vi "Flow Sensors Control.vi"(5 "Initialized Array Cluster":T3, 7 "Initialized Index":i32, 9 "Apply Savitsky-Golay?":bool, 11 "Slave Data Cluster":T1={"Current DoE"=[], "SSI 1 Flow Rate"=0.0, "SSI 2 Flow Rate"=0.0, "FLOM 1 Flow Rate"=0.0, "FLOM 2 Flow Rate"=0.0, "Pumps Running?"=FALSE, "Boolean 2"=FALSE, "Boolean 3"=FALSE, "Boolean 4"=FALSE, "At Equilibrium?"=FALSE, "Script Running?"=FALSE, "Current Script Iteration"=0.0, "Total Script Iterations"=0.0, "FLOM Pumps VISA"="COM2", "SSI 1 Pump VISA"="COM76", "SSI 2 Pump VISA"="COM74", "Huber Unistat VISA"="COM1", "SSI 3 Pump VISA"="COM76", "SSI 4 Pump VISA"="COM76", "SSI 4 Flow Rate"=0.0, "SSI 3 Flow Rate"=0.0, "Flow Meter 1 Rate "=0.0, "Flow Meter 2 Rate"=0.0, "Flow Meter 3 Rate"=0.0, "Flow Meter 4 Rate"=0.0, "SSI 1 Flow Setpoint"=0.0, "SSI 2 Flow Setpoint"=0.0, "SSI 3 Flow Setpoint"=0.0, "SSI 4 Flow Setpoint"=0.0, "Temperature Setpoint"=0.0, "Flow meter 3 COM"=17, "Flow meter 5 COM"=18, "Flow meter 4 COM"=19, "Flow meter 2 COM"=16, "Flow meter 1 COM"=15, "Unit"=enum."PSI", "Pressure COM"="COM6", "Julabo Setpoint"=0.0, "Julabo Control"=enum."Internal", "Overtemp"=50.0, "Subtemp"=-20.0, "HeatMax"=50, "CoolMax"=-100, "InternMax"=50.0, "InternMin"=0.0, "Upper Bandlimit"=100.0, "Lower Bandlimit"=0.0, "Julabo CF41 VISA"="COM3", "Xp (0.6K) Int"=0.6, "Tn (3s) Int"=3, "Tv (0s) Int"=0, "Dynamic (0: aperiodic) Int"=enum."aperiodic", "Xp (0.6K) Ext"=0.6, "Tn (3s) Ext"=3, "Tv (0s) Ext"=0, "XpU (0.6K) Ext"=0.6, "Julabo Serial Configuration"={"Baud Rate"=4800, "Parity"=2, "Data Bits"=7, "Stop Bits"=10, "Flow Control"=2}} {"Julabo Serial Configuration"."Flow Control" items=["None", "XON/XOFF", "RTS/CTS", "XON/XOFF & RTS/CTS", "DTR/DSR", "XON/XOFF & DTR/DSR"]; "Julabo Serial Configuration"."Stop Bits" items=["1.0"=10, "1.5"=15, "2.0"=20]; "Julabo Serial Configuration"."Data Bits" items=["7"=7, "8"=8]; "Julabo Serial Configuration"."Parity" items=["None", "Odd", "Even", "Mark", "Space"]; "Julabo Serial Configuration"."Baud Rate" items=["300"=300, "600"=600, "1200"=1200, "2400"=2400, "4800"=4800, "9600"=9600, "19200"=19200]; "XpU (0.6K) Ext" min=0.1 max=99.9; "Tv (0s) Ext" max=999; "Tn (3s) Ext" min=3 max=9999; "Xp (0.6K) Ext" min=0.1 max=99.9; "Tv (0s) Int" max=999; "Tn (3s) Int" min=3 max=9999; "Xp (0.6K) Int" min=0.1 max=99.9; "Lower Bandlimit" min=0.0 max=200.0; "Upper Bandlimit" min=0.0 max=200.0; "InternMin" format="%.2f"; "InternMax" format="%.2f"; "CoolMax" min=-100 max=0; "HeatMax" max=100; "Subtemp" format="%.2f"; "Overtemp" format="%.2f"; "Julabo Setpoint" format="%.2f"; "Current DoE" format="%0.3f"}) -> (1 "Flow Rate Data Out":cluster{dbl, dbl, dbl, dbl, dbl}, 2 "Numeric out":i32, 3 "Flow Rate Data Array Cluster Out":T3)   [LabVIEW 2015]
uses:
  --Controls and TypeDefs--/DoE_Control_Cluster.ctl
  <instrlib>/JULABO DeviceDriver/Examples/Julabo Serial Control.ctl
  <vilib>/ptbypt/NI_PtbyPt.lvlib
panel:
  # "Julabo"
  # "Limits"
  # "PID Control Parameters"
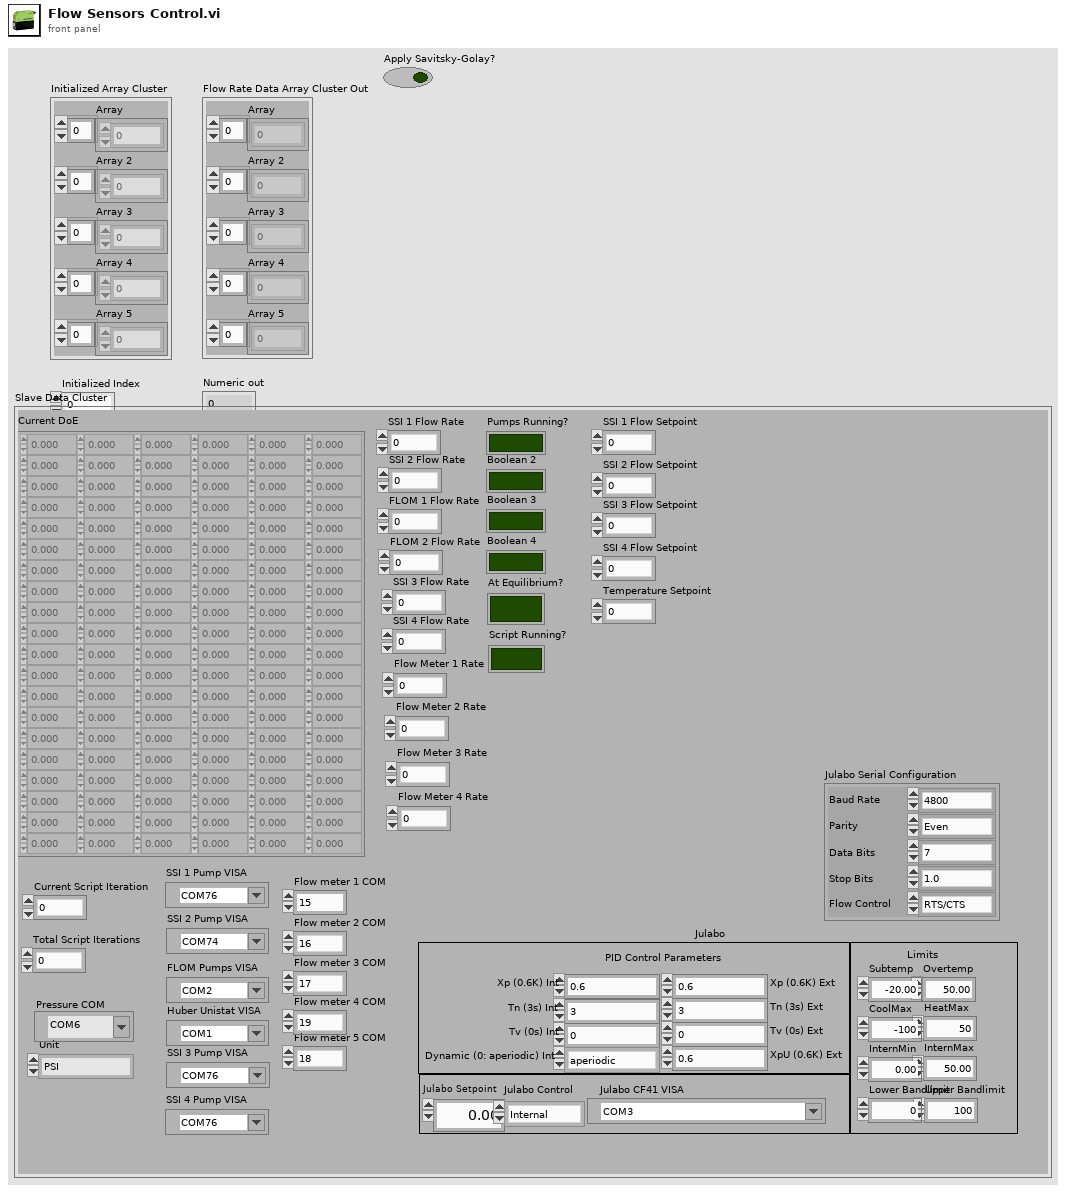
[diagram p1: front panel]
types:
  T1 = typedef "DoE_Control_Cluster.ctl" = cluster{"Current DoE":dbl[][], "SSI 1 Flow Rate":dbl, "SSI 2 Flow Rate":dbl, "FLOM 1 Flow Rate":dbl, "FLOM 2 Flow Rate":dbl, "Pumps Running?":bool, "Boolean 2":bool, "Boolean 3":bool, "Boolean 4":bool, "At Equilibrium?":bool, "Script Running?":bool, "Current Script Iteration":dbl, "Total Script Iterations":dbl, "FLOM Pumps VISA":refnum<visa-resource-name>, "SSI 1 Pump VISA":refnum<visa-resource-name>, "SSI 2 Pump VISA":refnum<visa-resource-name>, "Huber Unistat VISA":refnum<visa-resource-name>, "SSI 3 Pump VISA":refnum<visa-resource-name>, "SSI 4 Pump VISA":refnum<visa-resource-name>, "SSI 4 Flow Rate":dbl, "SSI 3 Flow Rate":dbl, "Flow Meter 1 Rate ":dbl, "Flow Meter 2 Rate":dbl, "Flow Meter 3 Rate":dbl, "Flow Meter 4 Rate":dbl, "SSI 1 Flow Setpoint":dbl, "SSI 2 Flow Setpoint":dbl, "SSI 3 Flow Setpoint":dbl, "SSI 4 Flow Setpoint":dbl, "Temperature Setpoint":dbl, "Flow meter 3 COM":u16, "Flow meter 5 COM":u16, "Flow meter 4 COM":u16, "Flow meter 2 COM":u16, "Flow meter 1 COM":u16, "Unit":enum16{"PSI", "Bar", "cm H2O", "ft H2O", "hectoPascal", "in Hg", "in H2O", "kiloPascal", "milliBar", "mmHg", "MegaPascal", "Numeric Pressure"}, "Pressure COM":refnum<visa-resource-name>, "Julabo Setpoint":dbl, "Julabo Control":enum16{"Internal", "External"}, "Overtemp":dbl, "Subtemp":dbl, "HeatMax":u8, "CoolMax":i8, "InternMax":dbl, "InternMin":dbl, "Upper Bandlimit":dbl, "Lower Bandlimit":dbl, "Julabo CF41 VISA":refnum<visa-resource-name>, "Xp (0.6K) Int":dbl, "Tn (3s) Int":u16, "Tv (0s) Int":u16, "Dynamic (0: aperiodic) Int":enum16{"aperiodic", "standard"}, "Xp (0.6K) Ext":dbl, "Tn (3s) Ext":u16, "Tv (0s) Ext":u16, "XpU (0.6K) Ext":dbl, "Julabo Serial Configuration":T2}
  T2 = typedef "Julabo Serial Control.ctl" = cluster{"Baud Rate":u32, "Parity":u16, "Data Bits":u16, "Stop Bits":u16, "Flow Control":u16}
  T3 = cluster{"Array":dbl[], "Array 2":dbl[], "Array 3":dbl[], "Array 4":dbl[], "Array 5":dbl[]}
  T4 = cluster{"Filtered x":dbl, "Filtered x":dbl, "Filtered x":dbl, "Filtered x":dbl, "Filtered x":dbl}
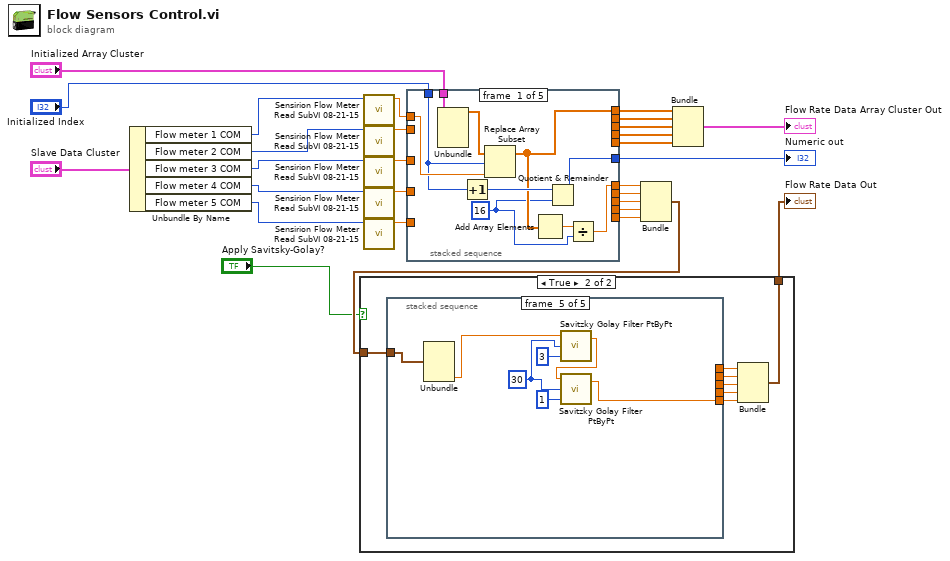
[diagram p0: block diagram]
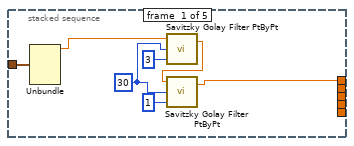
[diagram p3: hidden frame]
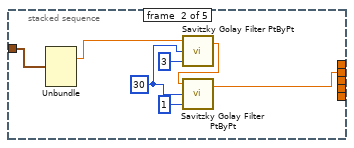
[diagram p4: hidden frame]
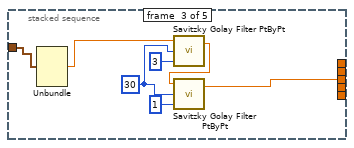
[diagram p5: hidden frame]
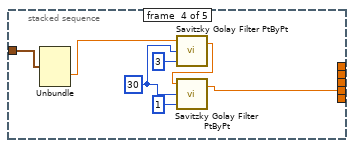
[diagram p6: hidden frame]
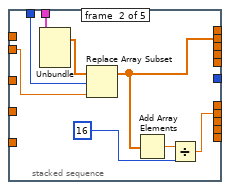
[diagram p7: hidden frame]
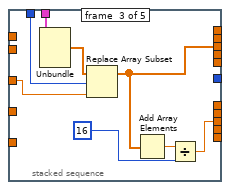
[diagram p8: hidden frame]
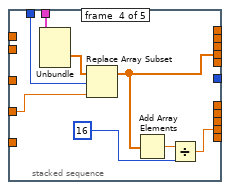
[diagram p9: hidden frame]
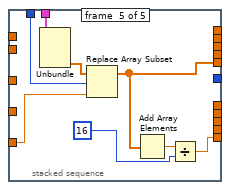
[diagram p10: hidden frame]
diagram:
  n1 = Unbundle By Name("Slave Data Cluster") -> ("Flow meter 1 COM"=w8:u16, "Flow meter 2 COM"=w7:u16, "Flow meter 3 COM"=w6:u16, "Flow meter 4 COM"=w5:u16, "Flow meter 5 COM"=w4:u16)
  n2 = call "Sensirion Flow Meter Read SubVI 08-21-15.vi"("COMPort"=w8) -> ("MeasureResult Scaled"=w10:dbl)  [unwired: 10 in]
  n3 = call "Sensirion Flow Meter Read SubVI 08-21-15.vi"("COMPort"=w7) -> ("MeasureResult Scaled"=w23:dbl)  [unwired: 10 in]
  n4 = call "Sensirion Flow Meter Read SubVI 08-21-15.vi"("COMPort"=w6) -> ("MeasureResult Scaled"=w24:dbl)  [unwired: 10 in]
  n5 = call "Sensirion Flow Meter Read SubVI 08-21-15.vi"("COMPort"=w5) -> ("MeasureResult Scaled"=w25:dbl)  [unwired: 10 in]
  n6 = call "Sensirion Flow Meter Read SubVI 08-21-15.vi"("COMPort"=w4) -> ("MeasureResult Scaled"=w26:dbl)  [unwired: 10 in]
  n7 = stacked-sequence {
    tunnel: [w34 _ _ _ _] -> w12
    tunnel: "Initialized Index" -> [w35 w46 w54 w62 w70]
    tunnel: [w37 _ _ _ _] -> w28
    tunnel: w10 -> [w36 _ _ _ _]
    tunnel: [w31 _ _ _ _] -> w11
    tunnel: "Initialized Array Cluster" -> [w30 w41 w51 w59 w67]
    tunnel: [_ w43 _ _ _] -> w13
    tunnel: [_ w42 _ _ _] -> w14
    tunnel: [_ _ w50 _ _] -> w17
    tunnel: [_ _ w49 _ _] -> w18
    tunnel: [_ _ _ w58 _] -> w19
    tunnel: [_ _ _ w57 _] -> w20
    tunnel: [_ _ _ _ w66] -> w21
    tunnel: [_ _ _ _ w64] -> w22
    tunnel: w23 -> [_ w39 _ _ _]
    tunnel: w24 -> [_ _ w47 _ _]
    tunnel: w25 -> [_ _ _ w55 _]
    tunnel: w26 -> [_ _ _ _ w63]
    frame #0 {
      w32 = 16 ("y")
      n8 = Unbundle(w30) -> ("Array"=w29:dbl[])  [unwired: 4 out]
      n9 = Increment(x=w35) -> (x+1=w38:i32)
      n10 = Replace Array Subset(array=w29, new element=w36, index=w35) -> (w34:dbl[])
      n11 = Add Array Elements(numeric array=w34) -> (sum=w33:dbl)
      n12 = Quotient & Remainder(x=w38, y=w32) -> (x-y*floor(x/y)=w37:i32)  [unwired: 1 out]
      n13 = Divide(x=w33, y=w32) -> (x/y=w31:dbl)
    }
    frame #1 {
      n14 = Unbundle(w41) -> ("Array 2"=w40:dbl[])  [unwired: 4 out]
      n15 = Replace Array Subset(array=w40, new element=w39, index=w46) -> (w42:dbl[])
      n16 = Add Array Elements(numeric array=w42) -> (sum=w45:dbl)
      n17 = Divide(x=w45, y=16) -> (x/y=w43:dbl)
    }
    frame #2 {
      n18 = Unbundle(w51) -> ("Array 3"=w48:dbl[])  [unwired: 4 out]
      n19 = Replace Array Subset(array=w48, new element=w47, index=w54) -> (w49:dbl[])
      n20 = Add Array Elements(numeric array=w49) -> (sum=w53:dbl)
      n21 = Divide(x=w53, y=16) -> (x/y=w50:dbl)
    }
    frame #3 {
      n22 = Unbundle(w59) -> ("Array 4"=w56:dbl[])  [unwired: 4 out]
      n23 = Replace Array Subset(array=w56, new element=w55, index=w62) -> (w58:dbl[])
      n24 = Add Array Elements(numeric array=w58) -> (sum=w61:dbl)
      n25 = Divide(x=w61, y=16) -> (x/y=w57:dbl)
    }
    frame #4 {
      n26 = Unbundle(w67) -> ("Array 5"=w65:dbl[])  [unwired: 4 out]
      n27 = Replace Array Subset(array=w65, new element=w63, index=w70) -> (w66:dbl[])
      n28 = Add Array Elements(numeric array=w66) -> (sum=w69:dbl)
      n29 = Divide(x=w69, y=16) -> (x/y=w64:dbl)
    }
  }
  "Numeric out" <- w28
  n30 = Bundle(w11, w13, w17, w20, w22) -> (w3:cluster{dbl, dbl, dbl, dbl, dbl})  [unwired: 1 in]
  n31 = case shown="True" "Apply Savitsky-Golay?" {
    tunnel: w3 -> [w71 w78]
    tunnel: [w71 w72] -> w2
    frame False {
    }
    frame True {
      n32 = stacked-sequence {
        tunnel: w78 -> [w85 w88 w95 w102 w109]
        tunnel: [w79 _ _ _ _] -> w77
        tunnel: [_ w86 _ _ _] -> w76
        tunnel: [_ _ w93 _ _] -> w75
        tunnel: [_ _ _ w100 _] -> w74
        tunnel: [_ _ _ _ w107] -> w73
        frame #0 {
          w80 = 30 ("side points")
          n33 = Unbundle(w85) -> (w82:dbl)  [unwired: 4 out]
          n34 = call <vilib>:"Savitzky Golay Filter PtByPt.vi"("order polynomial"=3 ("polynomial order"), "side points"=w80, "x"=w82) -> ("Filtered x"=w81:dbl)  [unwired: 1 in, 1 out]
          n35 = call <vilib>:"Savitzky Golay Filter PtByPt.vi"("order polynomial"=1 ("polynomial order"), "side points"=w80, "x"=w81) -> ("Filtered x"=w79:dbl)  [unwired: 1 in, 1 out]
        }
        frame #1 {
          w92 = 30 ("side points")
          n36 = Unbundle(w88) -> (w87:dbl)  [unwired: 4 out]
          n37 = call <vilib>:"Savitzky Golay Filter PtByPt.vi"("order polynomial"=3 ("polynomial order"), "side points"=w92, "x"=w87) -> ("Filtered x"=w91:dbl)  [unwired: 1 in, 1 out]
          n38 = call <vilib>:"Savitzky Golay Filter PtByPt.vi"("order polynomial"=1 ("polynomial order"), "side points"=w92, "x"=w91) -> ("Filtered x"=w86:dbl)  [unwired: 1 in, 1 out]
        }
        frame #2 {
          w96 = 30 ("side points")
          n39 = Unbundle(w95) -> (w94:dbl)  [unwired: 4 out]
          n40 = call <vilib>:"Savitzky Golay Filter PtByPt.vi"("order polynomial"=3 ("polynomial order"), "side points"=w96, "x"=w94) -> ("Filtered x"=w97:dbl)  [unwired: 1 in, 1 out]
          n41 = call <vilib>:"Savitzky Golay Filter PtByPt.vi"("order polynomial"=1 ("polynomial order"), "side points"=w96, "x"=w97) -> ("Filtered x"=w93:dbl)  [unwired: 1 in, 1 out]
        }
        frame #3 {
          w103 = 30 ("side points")
          n42 = Unbundle(w102) -> (w101:dbl)  [unwired: 4 out]
          n43 = call <vilib>:"Savitzky Golay Filter PtByPt.vi"("order polynomial"=3 ("polynomial order"), "side points"=w103, "x"=w101) -> ("Filtered x"=w104:dbl)  [unwired: 1 in, 1 out]
          n44 = call <vilib>:"Savitzky Golay Filter PtByPt.vi"("order polynomial"=1 ("polynomial order"), "side points"=w103, "x"=w104) -> ("Filtered x"=w100:dbl)  [unwired: 1 in, 1 out]
        }
        frame #4 {
          w110 = 30 ("side points")
          n45 = Unbundle(w109) -> (w108:dbl)  [unwired: 4 out]
          n46 = call <vilib>:"Savitzky Golay Filter PtByPt.vi"("order polynomial"=3 ("polynomial order"), "side points"=w110, "x"=w108) -> ("Filtered x"=w111:dbl)  [unwired: 1 in, 1 out]
          n47 = call <vilib>:"Savitzky Golay Filter PtByPt.vi"("order polynomial"=1 ("polynomial order"), "side points"=w110, "x"=w111) -> ("Filtered x"=w107:dbl)  [unwired: 1 in, 1 out]
        }
      }
      n48 = Bundle("Filtered x"=w77, "Filtered x"=w76, "Filtered x"=w75, "Filtered x"=w74, "Filtered x"=w73) -> (w72:T4)  [unwired: 1 in]
    }
  }
  "Flow Rate Data Out" <- w2
  n49 = Bundle("Array"=w12, "Array 2"=w14, "Array 3"=w18, "Array 4"=w19, "Array 5"=w21) -> (→"Flow Rate Data Array Cluster Out":T3)  [unwired: 1 in]
